vi "HandleObservationSync_002.vi"(8 "error in (no error)":errorcluster, 11 "S4GUI in":refnum<class "S4GUI.lvclass">) -> (0 "error out":errorcluster, 3 "S4GUI out":refnum<class "S4GUI.lvclass">)   [LabVIEW 2018, in "S4GUI.lvclass"] (continued)
          n492 = call-dynamic "Get CCD_Config.vi"("error in (no error)"=w1255, "Interface in"=w1261) -> ("error out"=w1268:errorcluster, "output cluster"=w1270:T1, "Interface out"=w1267:refnum<class "Interface.lvclass">)  [unwired: 7 in]
          n493 = Bundle By Name(cluster=w1270, "TRIGGER_MODE"=w1269) -> (w1266:T1)
          n494 = call-dynamic "Set CCD_Config.vi"("error in (no error)"=w1268, "input cluster"=w1266, "Interface in"=w1267) -> ("error out"=w1264:errorcluster, "Interface out"=w1262:refnum<class "Interface.lvclass">)  [unwired: 7 in]
          n495 = Flatten To String(anything=w1266, error in (no error)=w1264) -> (data string=w1265:string, error out=w1263:errorcluster)  [unwired: 2 in, 1 out]
          n496 = call "Write flatted cluster.vi"("error in (no error)"=w1263, "flatted cluster"=w1265, "Interface in"=w1262) -> ("error out"=w1258:errorcluster, "Interface out"=w1259:refnum<class "Interface.lvclass">)  [unwired: 7 in]
          n497 = Increment(x=w1295) -> (x+1=w1294:u32)
          n498 = call-dynamic "Write Interface.vi"("error in (no error)"=w1258, "Interface.lvclass"=w1259, "Channel in"=w1260) -> ("error out"=w1254:errorcluster, "Channel out"=w1253:refnum<class "Channel.lvclass">)  [unwired: 7 in]
          n499 = call-dynamic "Read State Machine.vi"("error in (no error)"=w1254, "Device in"=w1253) -> ("error out"=w1281:errorcluster, "State Machine.lvclass"=w1283:refnum<class "State Machine.lvclass">, "Device out"=w1279:refnum<class "Channel.lvclass">)  [unwired: 7 in]
          n500 = call "Next State.vi"("error in (no error)"=w1281, "New_State"=60, "State Machine in"=w1283) -> ("error out"=w1276:errorcluster, "State Machine out"=w1277:refnum<class "State Machine.lvclass">)  [unwired: 7 in]
          n501 = call-dynamic "Write State Machine.vi"("error in (no error)"=w1276, "State Machine.lvclass"=w1277, "Device in"=w1279) -> ("error out"=w1278:errorcluster, "Device out"=w1280:refnum<class "Channel.lvclass">)  [unwired: 7 in]
          n502 = call-dynamic "Write Channel.vi"("error in (no error)"=w1278, "Channel.lvclass"=w1280, "Acquisition in"=w1284) -> ("error out"=w1271:errorcluster, "Acquisition out"=w1272:refnum<class "Acquisition.lvclass">)  [unwired: 7 in]
          n503 = call-dynamic "Write AcquisitionA.vi"("error in (no error)"=w1271, "Acquisition.lvclass"=w1272, "S4ACS_GUI in"=w1273) -> ("error out"=w1286:errorcluster, "S4ACS_GUI out"=w1285:refnum<class "S4GUI.lvclass">)  [unwired: 7 in]
          n504 = Bundle By Name(cluster=w1285, "Obs_state"=w1294) -> (w1293:refnum<class "S4GUI.lvclass">)
        }
        frame 254 {
          # "Espera terminar a execução do comando atual \nantes de ir ao proximo passo da Observação."
          n505 = call-dynamic "Read AcquisitionA.vi"("error in (no error)"=w1315, "S4ACS_GUI in"=w1316) -> ("error out"=w1321:errorcluster, "Acquisition.lvclass"=w1322:refnum<class "Acquisition.lvclass">, "S4ACS_GUI out"=w1318:refnum<class "S4GUI.lvclass">)  [unwired: 7 in]
          n506 = call-dynamic "Read Channel.vi"("error in (no error)"=w1321, "Acquisition in"=w1322) -> ("error out"=w1313:errorcluster, "Channel.lvclass"=w1312:refnum<class "Channel.lvclass">, "Acquisition out"=w1320:refnum<class "Acquisition.lvclass">)  [unwired: 7 in]
          n507 = call-dynamic "Read State Machine.vi"("error in (no error)"=w1313, "Device in"=w1312) -> ("error out"=w1304:errorcluster, "State Machine.lvclass"=w1306:refnum<class "State Machine.lvclass">, "Device out"=w1310:refnum<class "Channel.lvclass">)  [unwired: 7 in]
          n508 = call-dynamic "Read State.vi"("error in (no error)"=w1304, "State Machine in"=w1306) -> ("error out"=w1303:errorcluster, "State"=w1300:i32, "State Machine out"=w1305:refnum<class "State Machine.lvclass">)  [unwired: 7 in]
          n509 = Equal To 0?(x=w1300) -> (x = 0?=w1302:bool)
          n510 = call-dynamic "Write State Machine.vi"("error in (no error)"=w1303, "State Machine.lvclass"=w1305, "Device in"=w1310) -> ("error out"=w1309:errorcluster, "Device out"=w1311:refnum<class "Channel.lvclass">)  [unwired: 7 in]
          n511 = call-dynamic "Write Channel.vi"("error in (no error)"=w1309, "Channel.lvclass"=w1311, "Acquisition in"=w1320) -> ("error out"=w1317:errorcluster, "Acquisition out"=w1319:refnum<class "Acquisition.lvclass">)  [unwired: 7 in]
          n512 = disable-structure shown="Enabled" {
            disable-tunnel: [u32 299 ("t") w1324] -> w1299
            disable-tunnel: w1298 -> [_ w1325]
            frame Disabled {
            }
            frame Enabled {
              n513 = Increment(x=w1325) -> (x+1=w1324:u32)
            }
          }
          n514 = Select(t=w1299, s=w1302, f=w1298) -> (s? t:f=w1301:u32)
          n515 = call-dynamic "Write AcquisitionA.vi"("error in (no error)"=w1317, "Acquisition.lvclass"=w1319, "S4ACS_GUI in"=w1318) -> ("error out"=w1314:errorcluster, "S4ACS_GUI out"=w1308:refnum<class "S4GUI.lvclass">)  [unwired: 7 in]
          n516 = Bundle By Name(cluster=w1308, "Obs_state"=w1301) -> (w1307:refnum<class "S4GUI.lvclass">)
        }
        frame 255 {
          n517 = call "Read AcquisitionB.vi"("error in (no error)"=w1336, "S4ACS_GUI in"=w1337) -> ("error out"=w1329:errorcluster, "Acquisition.lvclass"=w1330:refnum<class "Acquisition.lvclass">, "S4ACS_GUI out"=w1339:refnum<class "S4GUI.lvclass">)  [unwired: 7 in]
          n518 = call "Read connection.vi"("error in (no error)"=w1329, "Server in"=w1330) -> ("error out"=w1328:errorcluster, "connection"=w1326:bool, "Server out"=w1327:refnum<class "Acquisition.lvclass">)  [unwired: 7 in]
          n519 = case shown="False" w1326 {
            tunnel: w1327 -> [w1347 w1367]
            tunnel: w1328 -> [w1346 w1366]
            tunnel: [w1347 w1364] -> w1340
            tunnel: [w1346 w1363] -> w1338
            tunnel: w1333 -> [w1345 w1356]
            tunnel: [w1341 w1355] -> w1332
            frame False {
              n520 = Increment(x=w1345) -> (x+1=w1344:u32)
              n521 = Increment(x=w1344) -> (x+1=w1343:u32)
              n522 = Increment(x=w1343) -> (x+1=w1342:u32)
              n523 = Increment(x=w1342) -> (x+1=w1341:u32)
            }
            frame True {
              # "configura o canal,\nmas não dispara\na exposicao."
              n524 = call-dynamic "Read Channel.vi"("error in (no error)"=w1366, "Acquisition in"=w1367) -> ("error out"=w1352:errorcluster, "Channel.lvclass"=w1354:refnum<class "Channel.lvclass">, "Acquisition out"=w1365:refnum<class "Acquisition.lvclass">)  [unwired: 7 in]
              n525 = call-dynamic "Write expose.vi"("error in (no error)"=w1352, "expose"=FALSE, "Channel in"=w1354) -> ("error out"=w1351:errorcluster, "Channel out"=w1353:refnum<class "Channel.lvclass">)  [unwired: 7 in]
              n526 = call-dynamic "Read State Machine.vi"("error in (no error)"=w1351, "Device in"=w1353) -> ("error out"=w1360:errorcluster, "State Machine.lvclass"=w1362:refnum<class "State Machine.lvclass">, "Device out"=w1358:refnum<class "Channel.lvclass">)  [unwired: 7 in]
              n527 = call "Next State.vi"("error in (no error)"=w1360, "New_State"=1, "State Machine in"=w1362) -> ("error out"=w1348:errorcluster, "State Machine out"=w1349:refnum<class "State Machine.lvclass">)  [unwired: 7 in]
              n528 = Increment(x=w1356) -> (x+1=w1355:u32)
              n529 = call-dynamic "Write State Machine.vi"("error in (no error)"=w1348, "State Machine.lvclass"=w1349, "Device in"=w1358) -> ("error out"=w1357:errorcluster, "Device out"=w1359:refnum<class "Channel.lvclass">)  [unwired: 7 in]
              n530 = call-dynamic "Write Channel.vi"("error in (no error)"=w1357, "Channel.lvclass"=w1359, "Acquisition in"=w1365) -> ("error out"=w1363:errorcluster, "Acquisition out"=w1364:refnum<class "Acquisition.lvclass">)  [unwired: 7 in]
            }
          }
          n531 = call "Write AcquisitionB.vi"("error in (no error)"=w1338, "Acquisition.lvclass"=w1340, "S4ACS_GUI in"=w1339) -> ("error out"=w1335:errorcluster, "S4ACS_GUI out"=w1334:refnum<class "S4GUI.lvclass">)  [unwired: 7 in]
          n532 = Bundle By Name(cluster=w1334, "Obs_state"=w1332) -> (w1331:refnum<class "S4GUI.lvclass">)
        }
        frame 256 {
          # "Espera terminar a execução do comando atual \nantes de ir ao proximo passo da Observação."
          n533 = call "Read AcquisitionB.vi"("error in (no error)"=w1385, "S4ACS_GUI in"=w1386) -> ("error out"=w1391:errorcluster, "Acquisition.lvclass"=w1392:refnum<class "Acquisition.lvclass">, "S4ACS_GUI out"=w1388:refnum<class "S4GUI.lvclass">)  [unwired: 7 in]
          n534 = call-dynamic "Read Channel.vi"("error in (no error)"=w1391, "Acquisition in"=w1392) -> ("error out"=w1383:errorcluster, "Channel.lvclass"=w1382:refnum<class "Channel.lvclass">, "Acquisition out"=w1390:refnum<class "Acquisition.lvclass">)  [unwired: 7 in]
          n535 = call-dynamic "Read State Machine.vi"("error in (no error)"=w1383, "Device in"=w1382) -> ("error out"=w1374:errorcluster, "State Machine.lvclass"=w1376:refnum<class "State Machine.lvclass">, "Device out"=w1380:refnum<class "Channel.lvclass">)  [unwired: 7 in]
          n536 = call-dynamic "Read State.vi"("error in (no error)"=w1374, "State Machine in"=w1376) -> ("error out"=w1373:errorcluster, "State"=w1370:i32, "State Machine out"=w1375:refnum<class "State Machine.lvclass">)  [unwired: 7 in]
          n537 = call-dynamic "Write State Machine.vi"("error in (no error)"=w1373, "State Machine.lvclass"=w1375, "Device in"=w1380) -> ("error out"=w1379:errorcluster, "Device out"=w1381:refnum<class "Channel.lvclass">)  [unwired: 7 in]
          n538 = call-dynamic "Write Channel.vi"("error in (no error)"=w1379, "Channel.lvclass"=w1381, "Acquisition in"=w1390) -> ("error out"=w1387:errorcluster, "Acquisition out"=w1389:refnum<class "Acquisition.lvclass">)  [unwired: 7 in]
          n539 = Equal To 0?(x=w1370) -> (x = 0?=w1372:bool)
          n540 = disable-structure shown="Enabled" {
            disable-tunnel: [u32 299 ("t") w1394] -> w1368
            disable-tunnel: w1369 -> [_ w1397]
            frame Disabled {
            }
            frame Enabled {
              n541 = Increment(x=w1397) -> (x+1=w1396:u32)
              n542 = Increment(x=w1396) -> (x+1=w1395:u32)
              n543 = Increment(x=w1395) -> (x+1=w1394:u32)
            }
          }
          n544 = Select(t=w1368, s=w1372, f=w1369) -> (s? t:f=w1371:u32)
          n545 = call "Write AcquisitionB.vi"("error in (no error)"=w1387, "Acquisition.lvclass"=w1389, "S4ACS_GUI in"=w1388) -> ("error out"=w1384:errorcluster, "S4ACS_GUI out"=w1378:refnum<class "S4GUI.lvclass">)  [unwired: 7 in]
          n546 = Bundle By Name(cluster=w1378, "Obs_state"=w1371) -> (w1377:refnum<class "S4GUI.lvclass">)
        }
        frame 257 {
          # "Sem SyncBox, \ntrigger mode = 0 (internal)\nCom SyncBox\ntrigger mode = 6 (ext. start)"
          n547 = call-dynamic "Read Sync Box.lvclass.vi"("error in (no error)"=w1435, "SPARC4_AC in"=w1434) -> ("error out"=w1437:errorcluster, "Sync Box.lvclass"=w1438:refnum<class "Sync Box.lvclass">, "SPARC4_AC out"=w1433:refnum<class "S4GUI.lvclass">)  [unwired: 7 in]
          n548 = call "Read connection.vi"("error in (no error)"=w1437, "Server in"=w1438) -> ("error out"=w1436:errorcluster, "connection"=w1399:bool)  [unwired: 7 in, 1 out]
          n549 = case shown="False" w1399 {
            tunnel: [u8 6 ("TRIGGER_MODE") u8 0 ("TRIGGER_MODE")] -> w1398
            frame True {
            }
            frame False {
            }
          }
          n550 = call "Read AcquisitionB.vi"("error in (no error)"=w1436, "S4ACS_GUI in"=w1433) -> ("error out"=w1420:errorcluster, "Acquisition.lvclass"=w1421:refnum<class "Acquisition.lvclass">, "S4ACS_GUI out"=w1419:refnum<class "S4GUI.lvclass">)  [unwired: 7 in]
          n551 = call-dynamic "Read Channel.vi"("error in (no error)"=w1420, "Acquisition in"=w1421) -> ("error out"=w1404:errorcluster, "Channel.lvclass"=w1403:refnum<class "Channel.lvclass">, "Acquisition out"=w1430:refnum<class "Acquisition.lvclass">)  [unwired: 7 in]
          n552 = call-dynamic "Read Interface.vi"("error in (no error)"=w1404, "Channel in"=w1403) -> ("error out"=w1402:errorcluster, "Interface.lvclass"=w1408:refnum<class "Interface.lvclass">, "Channel out"=w1407:refnum<class "Channel.lvclass">)  [unwired: 7 in]
          n553 = call-dynamic "Get CCD_Config.vi"("error in (no error)"=w1402, "Interface in"=w1408) -> ("error out"=w1415:errorcluster, "output cluster"=w1416:T1, "Interface out"=w1414:refnum<class "Interface.lvclass">)  [unwired: 7 in]
          n554 = Bundle By Name(cluster=w1416, "TRIGGER_MODE"=w1398) -> (w1413:T1)
          n555 = call-dynamic "Set CCD_Config.vi"("error in (no error)"=w1415, "input cluster"=w1413, "Interface in"=w1414) -> ("error out"=w1411:errorcluster, "Interface out"=w1409:refnum<class "Interface.lvclass">)  [unwired: 7 in]
          n556 = Flatten To String(anything=w1413, error in (no error)=w1411) -> (data string=w1412:string, error out=w1410:errorcluster)  [unwired: 2 in, 1 out]
          n557 = call "Write flatted cluster.vi"("error in (no error)"=w1410, "flatted cluster"=w1412, "Interface in"=w1409) -> ("error out"=w1405:errorcluster, "Interface out"=w1406:refnum<class "Interface.lvclass">)  [unwired: 7 in]
          n558 = Increment(x=w1441) -> (x+1=w1440:u32)
          n559 = call-dynamic "Write Interface.vi"("error in (no error)"=w1405, "Interface.lvclass"=w1406, "Channel in"=w1407) -> ("error out"=w1401:errorcluster, "Channel out"=w1400:refnum<class "Channel.lvclass">)  [unwired: 7 in]
          n560 = call-dynamic "Read State Machine.vi"("error in (no error)"=w1401, "Device in"=w1400) -> ("error out"=w1427:errorcluster, "State Machine.lvclass"=w1429:refnum<class "State Machine.lvclass">, "Device out"=w1425:refnum<class "Channel.lvclass">)  [unwired: 7 in]
          n561 = call "Next State.vi"("error in (no error)"=w1427, "New_State"=60, "State Machine in"=w1429) -> ("error out"=w1422:errorcluster, "State Machine out"=w1423:refnum<class "State Machine.lvclass">)  [unwired: 7 in]
          n562 = call-dynamic "Write State Machine.vi"("error in (no error)"=w1422, "State Machine.lvclass"=w1423, "Device in"=w1425) -> ("error out"=w1424:errorcluster, "Device out"=w1426:refnum<class "Channel.lvclass">)  [unwired: 7 in]
          n563 = call-dynamic "Write Channel.vi"("error in (no error)"=w1424, "Channel.lvclass"=w1426, "Acquisition in"=w1430) -> ("error out"=w1417:errorcluster, "Acquisition out"=w1418:refnum<class "Acquisition.lvclass">)  [unwired: 7 in]
          n564 = call "Write AcquisitionB.vi"("error in (no error)"=w1417, "Acquisition.lvclass"=w1418, "S4ACS_GUI in"=w1419) -> ("error out"=w1432:errorcluster, "S4ACS_GUI out"=w1431:refnum<class "S4GUI.lvclass">)  [unwired: 7 in]
          n565 = Bundle By Name(cluster=w1431, "Obs_state"=w1440) -> (w1439:refnum<class "S4GUI.lvclass">)
        }
        frame 258 {
          # "Espera terminar a execução do comando atual \nantes de ir ao proximo passo da Observação."
          n566 = call "Read AcquisitionB.vi"("error in (no error)"=w1461, "S4ACS_GUI in"=w1462) -> ("error out"=w1467:errorcluster, "Acquisition.lvclass"=w1468:refnum<class "Acquisition.lvclass">, "S4ACS_GUI out"=w1464:refnum<class "S4GUI.lvclass">)  [unwired: 7 in]
          n567 = call-dynamic "Read Channel.vi"("error in (no error)"=w1467, "Acquisition in"=w1468) -> ("error out"=w1459:errorcluster, "Channel.lvclass"=w1458:refnum<class "Channel.lvclass">, "Acquisition out"=w1466:refnum<class "Acquisition.lvclass">)  [unwired: 7 in]
          n568 = call-dynamic "Read State Machine.vi"("error in (no error)"=w1459, "Device in"=w1458) -> ("error out"=w1450:errorcluster, "State Machine.lvclass"=w1452:refnum<class "State Machine.lvclass">, "Device out"=w1456:refnum<class "Channel.lvclass">)  [unwired: 7 in]
          n569 = call-dynamic "Read State.vi"("error in (no error)"=w1450, "State Machine in"=w1452) -> ("error out"=w1449:errorcluster, "State"=w1446:i32, "State Machine out"=w1451:refnum<class "State Machine.lvclass">)  [unwired: 7 in]
          n570 = call-dynamic "Write State Machine.vi"("error in (no error)"=w1449, "State Machine.lvclass"=w1451, "Device in"=w1456) -> ("error out"=w1455:errorcluster, "Device out"=w1457:refnum<class "Channel.lvclass">)  [unwired: 7 in]
          n571 = call-dynamic "Write Channel.vi"("error in (no error)"=w1455, "Channel.lvclass"=w1457, "Acquisition in"=w1466) -> ("error out"=w1463:errorcluster, "Acquisition out"=w1465:refnum<class "Acquisition.lvclass">)  [unwired: 7 in]
          n572 = Equal To 0?(x=w1446) -> (x = 0?=w1448:bool)
          n573 = Increment(x=w1445) -> (x+1=w1444:u32)
          n574 = Select(t=w1444, s=w1448, f=w1445) -> (s? t:f=w1447:u32)
          n575 = call "Write AcquisitionB.vi"("error in (no error)"=w1463, "Acquisition.lvclass"=w1465, "S4ACS_GUI in"=w1464) -> ("error out"=w1460:errorcluster, "S4ACS_GUI out"=w1454:refnum<class "S4GUI.lvclass">)  [unwired: 7 in]
          n576 = Bundle By Name(cluster=w1454, "Obs_state"=w1447) -> (w1453:refnum<class "S4GUI.lvclass">)
        }
        frame 259 {
          n577 = call-dynamic "Read AcquisitionC.vi"("error in (no error)"=w1479, "S4ACS_GUI in"=w1480) -> ("error out"=w1471:errorcluster, "Acquisition.lvclass"=w1473:refnum<class "Acquisition.lvclass">, "S4ACS_GUI out"=w1482:refnum<class "S4GUI.lvclass">)  [unwired: 7 in]
          n578 = call "Read connection.vi"("error in (no error)"=w1471, "Server in"=w1473) -> ("error out"=w1470:errorcluster, "connection"=w1469:bool, "Server out"=w1472:refnum<class "Acquisition.lvclass">)  [unwired: 7 in]
          n579 = case shown="True" w1469 {
            tunnel: w1472 -> [w1489 w1510]
            tunnel: w1470 -> [w1490 w1509]
            tunnel: [w1489 w1507] -> w1483
            tunnel: [w1490 w1506] -> w1481
            tunnel: w1476 -> [w1488 w1499]
            tunnel: [w1484 w1498] -> w1475
            frame False {
              n580 = Increment(x=w1488) -> (x+1=w1487:u32)
              n581 = Increment(x=w1487) -> (x+1=w1486:u32)
              n582 = Increment(x=w1486) -> (x+1=w1485:u32)
              n583 = Increment(x=w1485) -> (x+1=w1484:u32)
            }
            frame True {
              # "configura o canal,\nmas não dispara\na exposicao."
              n584 = call-dynamic "Read Channel.vi"("error in (no error)"=w1509, "Acquisition in"=w1510) -> ("error out"=w1495:errorcluster, "Channel.lvclass"=w1497:refnum<class "Channel.lvclass">, "Acquisition out"=w1508:refnum<class "Acquisition.lvclass">)  [unwired: 7 in]
              n585 = call-dynamic "Write expose.vi"("error in (no error)"=w1495, "expose"=FALSE, "Channel in"=w1497) -> ("error out"=w1494:errorcluster, "Channel out"=w1496:refnum<class "Channel.lvclass">)  [unwired: 7 in]
              n586 = call-dynamic "Read State Machine.vi"("error in (no error)"=w1494, "Device in"=w1496) -> ("error out"=w1503:errorcluster, "State Machine.lvclass"=w1505:refnum<class "State Machine.lvclass">, "Device out"=w1501:refnum<class "Channel.lvclass">)  [unwired: 7 in]
              n587 = call "Next State.vi"("error in (no error)"=w1503, "New_State"=1, "State Machine in"=w1505) -> ("error out"=w1491:errorcluster, "State Machine out"=w1492:refnum<class "State Machine.lvclass">)  [unwired: 7 in]
              n588 = Increment(x=w1499) -> (x+1=w1498:u32)
              n589 = call-dynamic "Write State Machine.vi"("error in (no error)"=w1491, "State Machine.lvclass"=w1492, "Device in"=w1501) -> ("error out"=w1500:errorcluster, "Device out"=w1502:refnum<class "Channel.lvclass">)  [unwired: 7 in]
              n590 = call-dynamic "Write Channel.vi"("error in (no error)"=w1500, "Channel.lvclass"=w1502, "Acquisition in"=w1508) -> ("error out"=w1506:errorcluster, "Acquisition out"=w1507:refnum<class "Acquisition.lvclass">)  [unwired: 7 in]
            }
          }
          n591 = call-dynamic "Write AcquisitionC.vi"("error in (no error)"=w1481, "Acquisition.lvclass"=w1483, "S4ACS_GUI in"=w1482) -> ("error out"=w1478:errorcluster, "S4ACS_GUI out"=w1477:refnum<class "S4GUI.lvclass">)  [unwired: 7 in]
          n592 = Bundle By Name(cluster=w1477, "Obs_state"=w1475) -> (w1474:refnum<class "S4GUI.lvclass">)
        }
        frame 260 {
          # "Espera terminar a execução do comando atual \nantes de ir ao proximo passo da Observação."
          n593 = call-dynamic "Read AcquisitionC.vi"("error in (no error)"=w1528, "S4ACS_GUI in"=w1529) -> ("error out"=w1534:errorcluster, "Acquisition.lvclass"=w1535:refnum<class "Acquisition.lvclass">, "S4ACS_GUI out"=w1531:refnum<class "S4GUI.lvclass">)  [unwired: 7 in]
          n594 = call-dynamic "Read Channel.vi"("error in (no error)"=w1534, "Acquisition in"=w1535) -> ("error out"=w1526:errorcluster, "Channel.lvclass"=w1525:refnum<class "Channel.lvclass">, "Acquisition out"=w1533:refnum<class "Acquisition.lvclass">)  [unwired: 7 in]
          n595 = call-dynamic "Read State Machine.vi"("error in (no error)"=w1526, "Device in"=w1525) -> ("error out"=w1517:errorcluster, "State Machine.lvclass"=w1519:refnum<class "State Machine.lvclass">, "Device out"=w1523:refnum<class "Channel.lvclass">)  [unwired: 7 in]
          n596 = call-dynamic "Read State.vi"("error in (no error)"=w1517, "State Machine in"=w1519) -> ("error out"=w1516:errorcluster, "State"=w1513:i32, "State Machine out"=w1518:refnum<class "State Machine.lvclass">)  [unwired: 7 in]
          n597 = Equal To 0?(x=w1513) -> (x = 0?=w1515:bool)
          n598 = call-dynamic "Write State Machine.vi"("error in (no error)"=w1516, "State Machine.lvclass"=w1518, "Device in"=w1523) -> ("error out"=w1522:errorcluster, "Device out"=w1524:refnum<class "Channel.lvclass">)  [unwired: 7 in]
          n599 = call-dynamic "Write Channel.vi"("error in (no error)"=w1522, "Channel.lvclass"=w1524, "Acquisition in"=w1533) -> ("error out"=w1530:errorcluster, "Acquisition out"=w1532:refnum<class "Acquisition.lvclass">)  [unwired: 7 in]
          n600 = disable-structure shown="Enabled" {
            disable-tunnel: [u32 299 ("t") w1537] -> w1511
            disable-tunnel: w1512 -> [_ w1540]
            frame Disabled {
            }
            frame Enabled {
              n601 = Increment(x=w1540) -> (x+1=w1539:u32)
              n602 = Increment(x=w1539) -> (x+1=w1538:u32)
              n603 = Increment(x=w1538) -> (x+1=w1537:u32)
            }
          }
          n604 = Select(t=w1511, s=w1515, f=w1512) -> (s? t:f=w1514:u32)
          n605 = call-dynamic "Write AcquisitionC.vi"("error in (no error)"=w1530, "Acquisition.lvclass"=w1532, "S4ACS_GUI in"=w1531) -> ("error out"=w1527:errorcluster, "S4ACS_GUI out"=w1521:refnum<class "S4GUI.lvclass">)  [unwired: 7 in]
          n606 = Bundle By Name(cluster=w1521, "Obs_state"=w1514) -> (w1520:refnum<class "S4GUI.lvclass">)
        }
        frame 261 {
          # "Sem SyncBox, \ntrigger mode = 0 (internal)\nCom SyncBox\ntrigger mode = 6 (ext. start)"
          n607 = call-dynamic "Read Sync Box.lvclass.vi"("error in (no error)"=w1578, "SPARC4_AC in"=w1577) -> ("error out"=w1580:errorcluster, "Sync Box.lvclass"=w1581:refnum<class "Sync Box.lvclass">, "SPARC4_AC out"=w1576:refnum<class "S4GUI.lvclass">)  [unwired: 7 in]
          n608 = call "Read connection.vi"("error in (no error)"=w1580, "Server in"=w1581) -> ("error out"=w1579:errorcluster, "connection"=w1542:bool)  [unwired: 7 in, 1 out]
          n609 = case shown="False" w1542 {
            tunnel: [u8 6 ("TRIGGER_MODE") u8 0 ("TRIGGER_MODE")] -> w1541
            frame True {
            }
            frame False {
            }
          }
          n610 = call-dynamic "Read AcquisitionC.vi"("error in (no error)"=w1579, "S4ACS_GUI in"=w1576) -> ("error out"=w1563:errorcluster, "Acquisition.lvclass"=w1564:refnum<class "Acquisition.lvclass">, "S4ACS_GUI out"=w1562:refnum<class "S4GUI.lvclass">)  [unwired: 7 in]
          n611 = call-dynamic "Read Channel.vi"("error in (no error)"=w1563, "Acquisition in"=w1564) -> ("error out"=w1547:errorcluster, "Channel.lvclass"=w1546:refnum<class "Channel.lvclass">, "Acquisition out"=w1573:refnum<class "Acquisition.lvclass">)  [unwired: 7 in]
          n612 = call-dynamic "Read Interface.vi"("error in (no error)"=w1547, "Channel in"=w1546) -> ("error out"=w1545:errorcluster, "Interface.lvclass"=w1551:refnum<class "Interface.lvclass">, "Channel out"=w1550:refnum<class "Channel.lvclass">)  [unwired: 7 in]
          n613 = call-dynamic "Get CCD_Config.vi"("error in (no error)"=w1545, "Interface in"=w1551) -> ("error out"=w1558:errorcluster, "output cluster"=w1559:T1, "Interface out"=w1557:refnum<class "Interface.lvclass">)  [unwired: 7 in]
          n614 = Bundle By Name(cluster=w1559, "TRIGGER_MODE"=w1541) -> (w1556:T1)
          n615 = call-dynamic "Set CCD_Config.vi"("error in (no error)"=w1558, "input cluster"=w1556, "Interface in"=w1557) -> ("error out"=w1554:errorcluster, "Interface out"=w1552:refnum<class "Interface.lvclass">)  [unwired: 7 in]
          n616 = Flatten To String(anything=w1556, error in (no error)=w1554) -> (data string=w1555:string, error out=w1553:errorcluster)  [unwired: 2 in, 1 out]
          n617 = call "Write flatted cluster.vi"("error in (no error)"=w1553, "flatted cluster"=w1555, "Interface in"=w1552) -> ("error out"=w1548:errorcluster, "Interface out"=w1549:refnum<class "Interface.lvclass">)  [unwired: 7 in]
          n618 = Increment(x=w1584) -> (x+1=w1583:u32)
          n619 = call-dynamic "Write Interface.vi"("error in (no error)"=w1548, "Interface.lvclass"=w1549, "Channel in"=w1550) -> ("error out"=w1544:errorcluster, "Channel out"=w1543:refnum<class "Channel.lvclass">)  [unwired: 7 in]
          n620 = call-dynamic "Read State Machine.vi"("error in (no error)"=w1544, "Device in"=w1543) -> ("error out"=w1570:errorcluster, "State Machine.lvclass"=w1572:refnum<class "State Machine.lvclass">, "Device out"=w1568:refnum<class "Channel.lvclass">)  [unwired: 7 in]
          n621 = call "Next State.vi"("error in (no error)"=w1570, "New_State"=60, "State Machine in"=w1572) -> ("error out"=w1565:errorcluster, "State Machine out"=w1566:refnum<class "State Machine.lvclass">)  [unwired: 7 in]
          n622 = call-dynamic "Write State Machine.vi"("error in (no error)"=w1565, "State Machine.lvclass"=w1566, "Device in"=w1568) -> ("error out"=w1567:errorcluster, "Device out"=w1569:refnum<class "Channel.lvclass">)  [unwired: 7 in]
          n623 = call-dynamic "Write Channel.vi"("error in (no error)"=w1567, "Channel.lvclass"=w1569, "Acquisition in"=w1573) -> ("error out"=w1560:errorcluster, "Acquisition out"=w1561:refnum<class "Acquisition.lvclass">)  [unwired: 7 in]
          n624 = call-dynamic "Write AcquisitionC.vi"("error in (no error)"=w1560, "Acquisition.lvclass"=w1561, "S4ACS_GUI in"=w1562) -> ("error out"=w1575:errorcluster, "S4ACS_GUI out"=w1574:refnum<class "S4GUI.lvclass">)  [unwired: 7 in]
          n625 = Bundle By Name(cluster=w1574, "Obs_state"=w1583) -> (w1582:refnum<class "S4GUI.lvclass">)
        }
        frame 262 {
          # "Espera terminar a execução do comando atual \nantes de ir ao proximo passo da Observação."
          n626 = call-dynamic "Read AcquisitionC.vi"("error in (no error)"=w1604, "S4ACS_GUI in"=w1605) -> ("error out"=w1610:errorcluster, "Acquisition.lvclass"=w1611:refnum<class "Acquisition.lvclass">, "S4ACS_GUI out"=w1607:refnum<class "S4GUI.lvclass">)  [unwired: 7 in]
          n627 = call-dynamic "Read Channel.vi"("error in (no error)"=w1610, "Acquisition in"=w1611) -> ("error out"=w1602:errorcluster, "Channel.lvclass"=w1601:refnum<class "Channel.lvclass">, "Acquisition out"=w1609:refnum<class "Acquisition.lvclass">)  [unwired: 7 in]
          n628 = call-dynamic "Read State Machine.vi"("error in (no error)"=w1602, "Device in"=w1601) -> ("error out"=w1593:errorcluster, "State Machine.lvclass"=w1595:refnum<class "State Machine.lvclass">, "Device out"=w1599:refnum<class "Channel.lvclass">)  [unwired: 7 in]
          n629 = call-dynamic "Read State.vi"("error in (no error)"=w1593, "State Machine in"=w1595) -> ("error out"=w1592:errorcluster, "State"=w1589:i32, "State Machine out"=w1594:refnum<class "State Machine.lvclass">)  [unwired: 7 in]
          n630 = Equal To 0?(x=w1589) -> (x = 0?=w1591:bool)
          n631 = call-dynamic "Write State Machine.vi"("error in (no error)"=w1592, "State Machine.lvclass"=w1594, "Device in"=w1599) -> ("error out"=w1598:errorcluster, "Device out"=w1600:refnum<class "Channel.lvclass">)  [unwired: 7 in]
          n632 = call-dynamic "Write Channel.vi"("error in (no error)"=w1598, "Channel.lvclass"=w1600, "Acquisition in"=w1609) -> ("error out"=w1606:errorcluster, "Acquisition out"=w1608:refnum<class "Acquisition.lvclass">)  [unwired: 7 in]
          n633 = Increment(x=w1588) -> (x+1=w1587:u32)
          n634 = Select(t=w1587, s=w1591, f=w1588) -> (s? t:f=w1590:u32)
          n635 = call-dynamic "Write AcquisitionC.vi"("error in (no error)"=w1606, "Acquisition.lvclass"=w1608, "S4ACS_GUI in"=w1607) -> ("error out"=w1603:errorcluster, "S4ACS_GUI out"=w1597:refnum<class "S4GUI.lvclass">)  [unwired: 7 in]
          n636 = Bundle By Name(cluster=w1597, "Obs_state"=w1590) -> (w1596:refnum<class "S4GUI.lvclass">)
        }
        frame 263 {
          # "Dispara o comando para o dispositivo corrente."
          n637 = call-dynamic "Read AcquisitionD.vi"("error in (no error)"=w1622, "S4ACS_GUI in"=w1623) -> ("error out"=w1615:errorcluster, "Acquisition.lvclass"=w1616:refnum<class "Acquisition.lvclass">, "S4ACS_GUI out"=w1625:refnum<class "S4GUI.lvclass">)  [unwired: 7 in]
          n638 = call "Read connection.vi"("error in (no error)"=w1615, "Server in"=w1616) -> ("error out"=w1613:errorcluster, "connection"=w1612:bool, "Server out"=w1614:refnum<class "Acquisition.lvclass">)  [unwired: 7 in]
          n639 = case shown="True" w1612 {
            tunnel: w1614 -> [w1629 w1649]
            tunnel: w1613 -> [w1628 w1648]
            tunnel: [w1629 w1646] -> w1626
            tunnel: [w1628 w1645] -> w1624
            tunnel: w1619 -> [_ w1638]
            tunnel: [u32 299 w1637] -> w1618
            frame False {
            }
            frame True {
              # "configura o canal,\nmas não dispara\na exposicao."
              n640 = call-dynamic "Read Channel.vi"("error in (no error)"=w1648, "Acquisition in"=w1649) -> ("error out"=w1634:errorcluster, "Channel.lvclass"=w1636:refnum<class "Channel.lvclass">, "Acquisition out"=w1647:refnum<class "Acquisition.lvclass">)  [unwired: 7 in]
              n641 = call-dynamic "Write expose.vi"("error in (no error)"=w1634, "expose"=FALSE, "Channel in"=w1636) -> ("error out"=w1633:errorcluster, "Channel out"=w1635:refnum<class "Channel.lvclass">)  [unwired: 7 in]
              n642 = call-dynamic "Read State Machine.vi"("error in (no error)"=w1633, "Device in"=w1635) -> ("error out"=w1642:errorcluster, "State Machine.lvclass"=w1644:refnum<class "State Machine.lvclass">, "Device out"=w1640:refnum<class "Channel.lvclass">)  [unwired: 7 in]
              n643 = call "Next State.vi"("error in (no error)"=w1642, "New_State"=1, "State Machine in"=w1644) -> ("error out"=w1630:errorcluster, "State Machine out"=w1631:refnum<class "State Machine.lvclass">)  [unwired: 7 in]
              n644 = Increment(x=w1638) -> (x+1=w1637:u32)
              n645 = call-dynamic "Write State Machine.vi"("error in (no error)"=w1630, "State Machine.lvclass"=w1631, "Device in"=w1640) -> ("error out"=w1639:errorcluster, "Device out"=w1641:refnum<class "Channel.lvclass">)  [unwired: 7 in]
              n646 = call-dynamic "Write Channel.vi"("error in (no error)"=w1639, "Channel.lvclass"=w1641, "Acquisition in"=w1647) -> ("error out"=w1645:errorcluster, "Acquisition out"=w1646:refnum<class "Acquisition.lvclass">)  [unwired: 7 in]
            }
          }
          n647 = call-dynamic "Write AcquisitionD.vi"("error in (no error)"=w1624, "Acquisition.lvclass"=w1626, "S4ACS_GUI in"=w1625) -> ("error out"=w1621:errorcluster, "S4ACS_GUI out"=w1620:refnum<class "S4GUI.lvclass">)  [unwired: 7 in]
          n648 = Bundle By Name(cluster=w1620, "Obs_state"=w1618) -> (w1617:refnum<class "S4GUI.lvclass">)
        }
        frame 264 {
          # "Espera terminar a execução do comando atual \nantes de ir ao proximo passo da Observação."
          n649 = call-dynamic "Read AcquisitionD.vi"("error in (no error)"=w1667, "S4ACS_GUI in"=w1668) -> ("error out"=w1673:errorcluster, "Acquisition.lvclass"=w1674:refnum<class "Acquisition.lvclass">, "S4ACS_GUI out"=w1670:refnum<class "S4GUI.lvclass">)  [unwired: 7 in]
          n650 = call-dynamic "Read Channel.vi"("error in (no error)"=w1673, "Acquisition in"=w1674) -> ("error out"=w1665:errorcluster, "Channel.lvclass"=w1664:refnum<class "Channel.lvclass">, "Acquisition out"=w1672:refnum<class "Acquisition.lvclass">)  [unwired: 7 in]
          n651 = call-dynamic "Read State Machine.vi"("error in (no error)"=w1665, "Device in"=w1664) -> ("error out"=w1656:errorcluster, "State Machine.lvclass"=w1658:refnum<class "State Machine.lvclass">, "Device out"=w1662:refnum<class "Channel.lvclass">)  [unwired: 7 in]
          n652 = call-dynamic "Read State.vi"("error in (no error)"=w1656, "State Machine in"=w1658) -> ("error out"=w1655:errorcluster, "State"=w1652:i32, "State Machine out"=w1657:refnum<class "State Machine.lvclass">)  [unwired: 7 in]
          n653 = Equal To 0?(x=w1652) -> (x = 0?=w1654:bool)
          n654 = call-dynamic "Write State Machine.vi"("error in (no error)"=w1655, "State Machine.lvclass"=w1657, "Device in"=w1662) -> ("error out"=w1661:errorcluster, "Device out"=w1663:refnum<class "Channel.lvclass">)  [unwired: 7 in]
          n655 = call-dynamic "Write Channel.vi"("error in (no error)"=w1661, "Channel.lvclass"=w1663, "Acquisition in"=w1672) -> ("error out"=w1669:errorcluster, "Acquisition out"=w1671:refnum<class "Acquisition.lvclass">)  [unwired: 7 in]
          n656 = disable-structure shown="Enabled" {
            disable-tunnel: w1651 -> [w1676 _]
            disable-tunnel: [w1675 u32 299] -> w1650
            frame Disabled {
              n657 = Increment(x=w1676) -> (x+1=w1675:u32)
            }
            frame Enabled {
            }
          }
          n658 = Select(t=w1650, s=w1654, f=w1651) -> (s? t:f=w1653:u32)
          n659 = call-dynamic "Write AcquisitionD.vi"("error in (no error)"=w1669, "Acquisition.lvclass"=w1671, "S4ACS_GUI in"=w1670) -> ("error out"=w1666:errorcluster, "S4ACS_GUI out"=w1660:refnum<class "S4GUI.lvclass">)  [unwired: 7 in]
          n660 = Bundle By Name(cluster=w1660, "Obs_state"=w1653) -> (w1659:refnum<class "S4GUI.lvclass">)
        }
        frame 265 {
          # "Sem SyncBox, \ntrigger mode = 0 (internal)\nCom SyncBox\ntrigger mode = 6 (ext. start)"
          n661 = call-dynamic "Read Sync Box.lvclass.vi"("error in (no error)"=w1715, "SPARC4_AC in"=w1714) -> ("error out"=w1717:errorcluster, "Sync Box.lvclass"=w1718:refnum<class "Sync Box.lvclass">, "SPARC4_AC out"=w1713:refnum<class "S4GUI.lvclass">)  [unwired: 7 in]
          n662 = call "Read connection.vi"("error in (no error)"=w1717, "Server in"=w1718) -> ("error out"=w1716:errorcluster, "connection"=w1679:bool)  [unwired: 7 in, 1 out]
          n663 = case shown="False" w1679 {
            tunnel: [u8 6 ("TRIGGER_MODE") u8 0 ("TRIGGER_MODE")] -> w1678
            frame True {
            }
            frame False {
            }
          }
          n664 = call-dynamic "Read AcquisitionD.vi"("error in (no error)"=w1716, "S4ACS_GUI in"=w1713) -> ("error out"=w1700:errorcluster, "Acquisition.lvclass"=w1701:refnum<class "Acquisition.lvclass">, "S4ACS_GUI out"=w1699:refnum<class "S4GUI.lvclass">)  [unwired: 7 in]
          n665 = call-dynamic "Read Channel.vi"("error in (no error)"=w1700, "Acquisition in"=w1701) -> ("error out"=w1684:errorcluster, "Channel.lvclass"=w1683:refnum<class "Channel.lvclass">, "Acquisition out"=w1710:refnum<class "Acquisition.lvclass">)  [unwired: 7 in]
          n666 = call-dynamic "Read Interface.vi"("error in (no error)"=w1684, "Channel in"=w1683) -> ("error out"=w1682:errorcluster, "Interface.lvclass"=w1688:refnum<class "Interface.lvclass">, "Channel out"=w1687:refnum<class "Channel.lvclass">)  [unwired: 7 in]
          n667 = call-dynamic "Get CCD_Config.vi"("error in (no error)"=w1682, "Interface in"=w1688) -> ("error out"=w1695:errorcluster, "output cluster"=w1696:T1, "Interface out"=w1694:refnum<class "Interface.lvclass">)  [unwired: 7 in]
          n668 = Bundle By Name(cluster=w1696, "TRIGGER_MODE"=w1678) -> (w1693:T1)
          n669 = call-dynamic "Set CCD_Config.vi"("error in (no error)"=w1695, "input cluster"=w1693, "Interface in"=w1694) -> ("error out"=w1691:errorcluster, "Interface out"=w1689:refnum<class "Interface.lvclass">)  [unwired: 7 in]
          n670 = Flatten To String(anything=w1693, error in (no error)=w1691) -> (data string=w1692:string, error out=w1690:errorcluster)  [unwired: 2 in, 1 out]
          n671 = call "Write flatted cluster.vi"("error in (no error)"=w1690, "flatted cluster"=w1692, "Interface in"=w1689) -> ("error out"=w1685:errorcluster, "Interface out"=w1686:refnum<class "Interface.lvclass">)  [unwired: 7 in]
          n672 = call-dynamic "Write Interface.vi"("error in (no error)"=w1685, "Interface.lvclass"=w1686, "Channel in"=w1687) -> ("error out"=w1681:errorcluster, "Channel out"=w1680:refnum<class "Channel.lvclass">)  [unwired: 7 in]
          n673 = call-dynamic "Read State Machine.vi"("error in (no error)"=w1681, "Device in"=w1680) -> ("error out"=w1707:errorcluster, "State Machine.lvclass"=w1709:refnum<class "State Machine.lvclass">, "Device out"=w1705:refnum<class "Channel.lvclass">)  [unwired: 7 in]
          n674 = Increment(x=w1721) -> (x+1=w1720:u32)
          n675 = call "Next State.vi"("error in (no error)"=w1707, "New_State"=60, "State Machine in"=w1709) -> ("error out"=w1702:errorcluster, "State Machine out"=w1703:refnum<class "State Machine.lvclass">)  [unwired: 7 in]
          n676 = call-dynamic "Write State Machine.vi"("error in (no error)"=w1702, "State Machine.lvclass"=w1703, "Device in"=w1705) -> ("error out"=w1704:errorcluster, "Device out"=w1706:refnum<class "Channel.lvclass">)  [unwired: 7 in]
          n677 = call-dynamic "Write Channel.vi"("error in (no error)"=w1704, "Channel.lvclass"=w1706, "Acquisition in"=w1710) -> ("error out"=w1697:errorcluster, "Acquisition out"=w1698:refnum<class "Acquisition.lvclass">)  [unwired: 7 in]
          n678 = call-dynamic "Write AcquisitionD.vi"("error in (no error)"=w1697, "Acquisition.lvclass"=w1698, "S4ACS_GUI in"=w1699) -> ("error out"=w1712:errorcluster, "S4ACS_GUI out"=w1711:refnum<class "S4GUI.lvclass">)  [unwired: 7 in]
          n679 = Bundle By Name(cluster=w1711, "Obs_state"=w1720) -> (w1719:refnum<class "S4GUI.lvclass">)
        }
        frame 266 {
          # "Espera terminar a execução do comando atual \nantes de ir ao proximo passo da Observação."
          n680 = call-dynamic "Read AcquisitionD.vi"("error in (no error)"=w1741, "S4ACS_GUI in"=w1742) -> ("error out"=w1747:errorcluster, "Acquisition.lvclass"=w1748:refnum<class "Acquisition.lvclass">, "S4ACS_GUI out"=w1744:refnum<class "S4GUI.lvclass">)  [unwired: 7 in]
          n681 = call-dynamic "Read Channel.vi"("error in (no error)"=w1747, "Acquisition in"=w1748) -> ("error out"=w1739:errorcluster, "Channel.lvclass"=w1738:refnum<class "Channel.lvclass">, "Acquisition out"=w1746:refnum<class "Acquisition.lvclass">)  [unwired: 7 in]
          n682 = call-dynamic "Read State Machine.vi"("error in (no error)"=w1739, "Device in"=w1738) -> ("error out"=w1730:errorcluster, "State Machine.lvclass"=w1732:refnum<class "State Machine.lvclass">, "Device out"=w1736:refnum<class "Channel.lvclass">)  [unwired: 7 in]
          n683 = call-dynamic "Read State.vi"("error in (no error)"=w1730, "State Machine in"=w1732) -> ("error out"=w1729:errorcluster, "State"=w1726:i32, "State Machine out"=w1731:refnum<class "State Machine.lvclass">)  [unwired: 7 in]
          n684 = Equal To 0?(x=w1726) -> (x = 0?=w1728:bool)
          n685 = call-dynamic "Write State Machine.vi"("error in (no error)"=w1729, "State Machine.lvclass"=w1731, "Device in"=w1736) -> ("error out"=w1735:errorcluster, "Device out"=w1737:refnum<class "Channel.lvclass">)  [unwired: 7 in]
          n686 = call-dynamic "Write Channel.vi"("error in (no error)"=w1735, "Channel.lvclass"=w1737, "Acquisition in"=w1746) -> ("error out"=w1743:errorcluster, "Acquisition out"=w1745:refnum<class "Acquisition.lvclass">)  [unwired: 7 in]
          n687 = Select(t=u32 299, s=w1728, f=w1725) -> (s? t:f=w1727:u32)
          n688 = call-dynamic "Write AcquisitionD.vi"("error in (no error)"=w1743, "Acquisition.lvclass"=w1745, "S4ACS_GUI in"=w1744) -> ("error out"=w1740:errorcluster, "S4ACS_GUI out"=w1734:refnum<class "S4GUI.lvclass">)  [unwired: 7 in]
          n689 = Bundle By Name(cluster=w1734, "Obs_state"=w1727) -> (w1733:refnum<class "S4GUI.lvclass">)
        }
        frame 271 {
          # "Prepara os canais de aquisição para sequencia de foco...."
          n690 = flat-sequence {
            tunnel: w1775 -> [w1880]
            tunnel: [w1880] -> w1774
            frame #0 {
              n691 = Tick Count (ms)() -> (millisecond timer value=→"time5":u32)
            }
          }
          n692 = call-dynamic "Read AcquisitionA.vi"("error in (no error)"=w1774, "S4ACS_GUI in"=w1796) -> ("error out"=w1794:errorcluster, "Acquisition.lvclass"=w1795:refnum<class "Acquisition.lvclass">, "S4ACS_GUI out"=w1798:refnum<class "S4GUI.lvclass">)  [unwired: 7 in]
          n693 = call "Read connection.vi"("error in (no error)"=w1794, "Server in"=w1795) -> ("error out"=w1793:errorcluster, "connection"=w1773:bool, "Server out"=w1792:refnum<class "Acquisition.lvclass">)  [unwired: 7 in]
          n694 = case shown="True" w1773 {
            tunnel: [w1861 w1879] -> w1799
            tunnel: [w1860 w1878] -> w1797
            tunnel: w1793 -> [w1860 w1877]
            tunnel: w1792 -> [w1861 w1876]
            frame False {
            }
            frame True {
              # "configura o canal,\nmas não dispara\na exposicao."
              n695 = call-dynamic "Read Channel.vi"("error in (no error)"=w1877, "Acquisition in"=w1876) -> ("error out"=w1866:errorcluster, "Channel.lvclass"=w1868:refnum<class "Channel.lvclass">, "Acquisition out"=w1875:refnum<class "Acquisition.lvclass">)  [unwired: 7 in]
              n696 = call-dynamic "Write expose.vi"("error in (no error)"=w1866, "expose"=FALSE, "Channel in"=w1868) -> ("error out"=w1865:errorcluster, "Channel out"=w1867:refnum<class "Channel.lvclass">)  [unwired: 7 in]
              n697 = call-dynamic "Read State Machine.vi"("error in (no error)"=w1865, "Device in"=w1867) -> ("error out"=w1872:errorcluster, "State Machine.lvclass"=w1874:refnum<class "State Machine.lvclass">, "Device out"=w1870:refnum<class "Channel.lvclass">)  [unwired: 7 in]
              n698 = call "Next State.vi"("error in (no error)"=w1872, "New_State"=1, "State Machine in"=w1874) -> ("error out"=w1862:errorcluster, "State Machine out"=w1863:refnum<class "State Machine.lvclass">)  [unwired: 7 in]
              n699 = call-dynamic "Write State Machine.vi"("error in (no error)"=w1862, "State Machine.lvclass"=w1863, "Device in"=w1870) -> ("error out"=w1869:errorcluster, "Device out"=w1871:refnum<class "Channel.lvclass">)  [unwired: 7 in]
              n700 = call-dynamic "Write Channel.vi"("error in (no error)"=w1869, "Channel.lvclass"=w1871, "Acquisition in"=w1875) -> ("error out"=w1878:errorcluster, "Acquisition out"=w1879:refnum<class "Acquisition.lvclass">)  [unwired: 7 in]
            }
          }
          n701 = Increment(x=w1791) -> (x+1=w1755:u32)
          n702 = call-dynamic "Write AcquisitionA.vi"("error in (no error)"=w1797, "Acquisition.lvclass"=w1799, "S4ACS_GUI in"=w1798) -> ("error out"=w1787:errorcluster, "S4ACS_GUI out"=w1786:refnum<class "S4GUI.lvclass">)  [unwired: 7 in]
          n703 = call "Read AcquisitionB.vi"("error in (no error)"=w1787, "S4ACS_GUI in"=w1786) -> ("error out"=w1788:errorcluster, "Acquisition.lvclass"=w1789:refnum<class "Acquisition.lvclass">, "S4ACS_GUI out"=w1790:refnum<class "S4GUI.lvclass">)  [unwired: 7 in]
          n704 = call "Read connection.vi"("error in (no error)"=w1788, "Server in"=w1789) -> ("error out"=w1771:errorcluster, "connection"=w1770:bool, "Server out"=w1772:refnum<class "Acquisition.lvclass">)  [unwired: 7 in]
          n705 = case shown="True" w1770 {
            tunnel: [w1841 w1859] -> w1769
            tunnel: [w1840 w1858] -> w1768
            tunnel: w1771 -> [w1840 w1857]
            tunnel: w1772 -> [w1841 w1856]
            frame False {
            }
            frame True {
              # "configura o canal,\nmas não dispara\na exposicao."
              n706 = call-dynamic "Read Channel.vi"("error in (no error)"=w1857, "Acquisition in"=w1856) -> ("error out"=w1846:errorcluster, "Channel.lvclass"=w1848:refnum<class "Channel.lvclass">, "Acquisition out"=w1855:refnum<class "Acquisition.lvclass">)  [unwired: 7 in]
              n707 = call-dynamic "Write expose.vi"("error in (no error)"=w1846, "expose"=FALSE, "Channel in"=w1848) -> ("error out"=w1845:errorcluster, "Channel out"=w1847:refnum<class "Channel.lvclass">)  [unwired: 7 in]
              n708 = call-dynamic "Read State Machine.vi"("error in (no error)"=w1845, "Device in"=w1847) -> ("error out"=w1852:errorcluster, "State Machine.lvclass"=w1854:refnum<class "State Machine.lvclass">, "Device out"=w1850:refnum<class "Channel.lvclass">)  [unwired: 7 in]
              n709 = call "Next State.vi"("error in (no error)"=w1852, "New_State"=1, "State Machine in"=w1854) -> ("error out"=w1842:errorcluster, "State Machine out"=w1843:refnum<class "State Machine.lvclass">)  [unwired: 7 in]
              n710 = call-dynamic "Write State Machine.vi"("error in (no error)"=w1842, "State Machine.lvclass"=w1843, "Device in"=w1850) -> ("error out"=w1849:errorcluster, "Device out"=w1851:refnum<class "Channel.lvclass">)  [unwired: 7 in]
              n711 = call-dynamic "Write Channel.vi"("error in (no error)"=w1849, "Channel.lvclass"=w1851, "Acquisition in"=w1855) -> ("error out"=w1858:errorcluster, "Acquisition out"=w1859:refnum<class "Acquisition.lvclass">)  [unwired: 7 in]
            }
          }
          n712 = call "Write AcquisitionB.vi"("error in (no error)"=w1768, "Acquisition.lvclass"=w1769, "S4ACS_GUI in"=w1790) -> ("error out"=w1779:errorcluster, "S4ACS_GUI out"=w1778:refnum<class "S4GUI.lvclass">)  [unwired: 7 in]
          n713 = call-dynamic "Read AcquisitionC.vi"("error in (no error)"=w1779, "S4ACS_GUI in"=w1778) -> ("error out"=w1783:errorcluster, "Acquisition.lvclass"=w1784:refnum<class "Acquisition.lvclass">, "S4ACS_GUI out"=w1785:refnum<class "S4GUI.lvclass">)  [unwired: 7 in]
          n714 = call "Read connection.vi"("error in (no error)"=w1783, "Server in"=w1784) -> ("error out"=w1765:errorcluster, "connection"=w1766:bool, "Server out"=w1767:refnum<class "Acquisition.lvclass">)  [unwired: 7 in]
          n715 = case shown="True" w1766 {
            tunnel: [w1821 w1839] -> w1764
            tunnel: [w1820 w1838] -> w1763
            tunnel: w1765 -> [w1820 w1837]
            tunnel: w1767 -> [w1821 w1836]
            frame False {
            }
            frame True {
              # "configura o canal,\nmas não dispara\na exposicao."
              n716 = call-dynamic "Read Channel.vi"("error in (no error)"=w1837, "Acquisition in"=w1836) -> ("error out"=w1826:errorcluster, "Channel.lvclass"=w1828:refnum<class "Channel.lvclass">, "Acquisition out"=w1835:refnum<class "Acquisition.lvclass">)  [unwired: 7 in]
              n717 = call-dynamic "Write expose.vi"("error in (no error)"=w1826, "expose"=FALSE, "Channel in"=w1828) -> ("error out"=w1825:errorcluster, "Channel out"=w1827:refnum<class "Channel.lvclass">)  [unwired: 7 in]
              n718 = call-dynamic "Read State Machine.vi"("error in (no error)"=w1825, "Device in"=w1827) -> ("error out"=w1832:errorcluster, "State Machine.lvclass"=w1834:refnum<class "State Machine.lvclass">, "Device out"=w1830:refnum<class "Channel.lvclass">)  [unwired: 7 in]
              n719 = call "Next State.vi"("error in (no error)"=w1832, "New_State"=1, "State Machine in"=w1834) -> ("error out"=w1822:errorcluster, "State Machine out"=w1823:refnum<class "State Machine.lvclass">)  [unwired: 7 in]
              n720 = call-dynamic "Write State Machine.vi"("error in (no error)"=w1822, "State Machine.lvclass"=w1823, "Device in"=w1830) -> ("error out"=w1829:errorcluster, "Device out"=w1831:refnum<class "Channel.lvclass">)  [unwired: 7 in]
              n721 = call-dynamic "Write Channel.vi"("error in (no error)"=w1829, "Channel.lvclass"=w1831, "Acquisition in"=w1835) -> ("error out"=w1838:errorcluster, "Acquisition out"=w1839:refnum<class "Acquisition.lvclass">)  [unwired: 7 in]
            }
          }
          n722 = call-dynamic "Write AcquisitionC.vi"("error in (no error)"=w1763, "Acquisition.lvclass"=w1764, "S4ACS_GUI in"=w1785) -> ("error out"=w1777:errorcluster, "S4ACS_GUI out"=w1776:refnum<class "S4GUI.lvclass">)  [unwired: 7 in]
          n723 = call-dynamic "Read AcquisitionD.vi"("error in (no error)"=w1777, "S4ACS_GUI in"=w1776) -> ("error out"=w1780:errorcluster, "Acquisition.lvclass"=w1781:refnum<class "Acquisition.lvclass">, "S4ACS_GUI out"=w1782:refnum<class "S4GUI.lvclass">)  [unwired: 7 in]
          n724 = call "Read connection.vi"("error in (no error)"=w1780, "Server in"=w1781) -> ("error out"=w1760:errorcluster, "connection"=w1762:bool, "Server out"=w1761:refnum<class "Acquisition.lvclass">)  [unwired: 7 in]
          n725 = case shown="True" w1762 {
            tunnel: [w1801 w1819] -> w1759
            tunnel: [w1800 w1818] -> w1758
            tunnel: w1760 -> [w1800 w1817]
            tunnel: w1761 -> [w1801 w1816]
            frame False {
            }
            frame True {
              # "configura o canal,\nmas não dispara\na exposicao."
              n726 = call-dynamic "Read Channel.vi"("error in (no error)"=w1817, "Acquisition in"=w1816) -> ("error out"=w1806:errorcluster, "Channel.lvclass"=w1808:refnum<class "Channel.lvclass">, "Acquisition out"=w1815:refnum<class "Acquisition.lvclass">)  [unwired: 7 in]
              n727 = call-dynamic "Write expose.vi"("error in (no error)"=w1806, "expose"=FALSE, "Channel in"=w1808) -> ("error out"=w1805:errorcluster, "Channel out"=w1807:refnum<class "Channel.lvclass">)  [unwired: 7 in]
              n728 = call-dynamic "Read State Machine.vi"("error in (no error)"=w1805, "Device in"=w1807) -> ("error out"=w1812:errorcluster, "State Machine.lvclass"=w1814:refnum<class "State Machine.lvclass">, "Device out"=w1810:refnum<class "Channel.lvclass">)  [unwired: 7 in]
              n729 = call "Next State.vi"("error in (no error)"=w1812, "New_State"=1, "State Machine in"=w1814) -> ("error out"=w1802:errorcluster, "State Machine out"=w1803:refnum<class "State Machine.lvclass">)  [unwired: 7 in]
              n730 = call-dynamic "Write State Machine.vi"("error in (no error)"=w1802, "State Machine.lvclass"=w1803, "Device in"=w1810) -> ("error out"=w1809:errorcluster, "Device out"=w1811:refnum<class "Channel.lvclass">)  [unwired: 7 in]
              n731 = call-dynamic "Write Channel.vi"("error in (no error)"=w1809, "Channel.lvclass"=w1811, "Acquisition in"=w1815) -> ("error out"=w1818:errorcluster, "Acquisition out"=w1819:refnum<class "Acquisition.lvclass">)  [unwired: 7 in]
            }
          }
          n732 = call-dynamic "Write AcquisitionD.vi"("error in (no error)"=w1758, "Acquisition.lvclass"=w1759, "S4ACS_GUI in"=w1782) -> ("error out"=w1750:errorcluster, "S4ACS_GUI out"=w1754:refnum<class "S4GUI.lvclass">)  [unwired: 7 in]
          n733 = Unbundle By Name(w1754) -> ("TelFocus.lvclass"=w1753:refnum<class "TelFocus.lvclass">)
          n734 = call-dynamic "Write focus #stepsdone.vi"("error in (no error)"=w1750, "focus #stepsdone"=u32 0, "TelFocus in"=w1753) -> ("error out"=w1749:errorcluster, "TelFocus out"=w1751:refnum<class "TelFocus.lvclass">)  [unwired: 7 in]
          n735 = Bundle By Name(cluster=w1754, "TelFocus.lvclass"=w1751, "Error Msg"="", "Obs_state"=w1755) -> (w1756:refnum<class "S4GUI.lvclass">)
        }
        frame 272 {
          w1890 = 38 ("x")
          w1899 = 28 ("x")
          # "Se algum canal foi pra 38: Texp inválido \npara a configuração do CCD."
          # "Se algum canal foi pra 28: ERRO na inicialização."
          # "Espera terminar a execução da preparação\ndos 4 canais antes de ir ao proximo passo \nda Observação."
          n736 = flat-sequence {
            tunnel: w1932 -> [w2037]
            tunnel: [w2037] -> w1931
            frame #0 {
              n737 = Tick Count (ms)() -> (millisecond timer value=→"time6":u32)
            }
          }
          n738 = call-dynamic "Read AcquisitionA.vi"("error in (no error)"=w1931, "S4ACS_GUI in"=w1942) -> ("error out"=w1929:errorcluster, "Acquisition.lvclass"=w1930:refnum<class "Acquisition.lvclass">, "S4ACS_GUI out"=w1944:refnum<class "S4GUI.lvclass">)  [unwired: 7 in]
          n739 = call "Read connection.vi"("error in (no error)"=w1929, "Server in"=w1930) -> ("error out"=w1927:errorcluster, "connection"=w1926:bool, "Server out"=w1928:refnum<class "Acquisition.lvclass">)  [unwired: 7 in]
          n740 = case shown="True" w1926 {
            tunnel: w1928 -> [w2020 w2036]
            tunnel: w1927 -> [w2019 w2035]
            tunnel: [w2020 w2033] -> w1945
            tunnel: [w2019 w2032] -> w1943
            tunnel: [0 ("State") w2022] -> w1889
            frame False {
            }
            frame True {
              n741 = call-dynamic "Read Channel.vi"("error in (no error)"=w2035, "Acquisition in"=w2036) -> ("error out"=w2031:errorcluster, "Channel.lvclass"=w2030:refnum<class "Channel.lvclass">, "Acquisition out"=w2034:refnum<class "Acquisition.lvclass">)  [unwired: 7 in]
              n742 = call-dynamic "Read State Machine.vi"("error in (no error)"=w2031, "Device in"=w2030) -> ("error out"=w2024:errorcluster, "State Machine.lvclass"=w2026:refnum<class "State Machine.lvclass">, "Device out"=w2028:refnum<class "Channel.lvclass">)  [unwired: 7 in]
              n743 = call-dynamic "Read State.vi"("error in (no error)"=w2024, "State Machine in"=w2026) -> ("error out"=w2023:errorcluster, "State"=w2022:i32, "State Machine out"=w2025:refnum<class "State Machine.lvclass">)  [unwired: 7 in]
              n744 = call-dynamic "Write State Machine.vi"("error in (no error)"=w2023, "State Machine.lvclass"=w2025, "Device in"=w2028) -> ("error out"=w2027:errorcluster, "Device out"=w2029:refnum<class "Channel.lvclass">)  [unwired: 7 in]
              n745 = call-dynamic "Write Channel.vi"("error in (no error)"=w2027, "Channel.lvclass"=w2029, "Acquisition in"=w2034) -> ("error out"=w2032:errorcluster, "Acquisition out"=w2033:refnum<class "Acquisition.lvclass">)  [unwired: 7 in]
            }
          }
          n746 = call-dynamic "Write AcquisitionA.vi"("error in (no error)"=w1943, "Acquisition.lvclass"=w1945, "S4ACS_GUI in"=w1944) -> ("error out"=w1939:errorcluster, "S4ACS_GUI out"=w1938:refnum<class "S4GUI.lvclass">)  [unwired: 7 in]
          n747 = call "Read AcquisitionB.vi"("error in (no error)"=w1939, "S4ACS_GUI in"=w1938) -> ("error out"=w1921:errorcluster, "Acquisition.lvclass"=w1924:refnum<class "Acquisition.lvclass">, "S4ACS_GUI out"=w1925:refnum<class "S4GUI.lvclass">)  [unwired: 7 in]
          n748 = call "Read connection.vi"("error in (no error)"=w1921, "Server in"=w1924) -> ("error out"=w1920:errorcluster, "connection"=w1922:bool, "Server out"=w1923:refnum<class "Acquisition.lvclass">)  [unwired: 7 in]
          n749 = case shown="True" w1922 {
            tunnel: w1923 -> [w2002 w2018]
            tunnel: w1920 -> [w2001 w2017]
            tunnel: [w2002 w2015] -> w1919
            tunnel: [w2001 w2014] -> w1918
            tunnel: [0 ("State") w2004] -> w1888
            frame False {
            }
            frame True {
              n750 = call-dynamic "Read Channel.vi"("error in (no error)"=w2017, "Acquisition in"=w2018) -> ("error out"=w2013:errorcluster, "Channel.lvclass"=w2012:refnum<class "Channel.lvclass">, "Acquisition out"=w2016:refnum<class "Acquisition.lvclass">)  [unwired: 7 in]
              n751 = call-dynamic "Read State Machine.vi"("error in (no error)"=w2013, "Device in"=w2012) -> ("error out"=w2006:errorcluster, "State Machine.lvclass"=w2008:refnum<class "State Machine.lvclass">, "Device out"=w2010:refnum<class "Channel.lvclass">)  [unwired: 7 in]
              n752 = call-dynamic "Read State.vi"("error in (no error)"=w2006, "State Machine in"=w2008) -> ("error out"=w2005:errorcluster, "State"=w2004:i32, "State Machine out"=w2007:refnum<class "State Machine.lvclass">)  [unwired: 7 in]
              n753 = call-dynamic "Write State Machine.vi"("error in (no error)"=w2005, "State Machine.lvclass"=w2007, "Device in"=w2010) -> ("error out"=w2009:errorcluster, "Device out"=w2011:refnum<class "Channel.lvclass">)  [unwired: 7 in]
              n754 = call-dynamic "Write Channel.vi"("error in (no error)"=w2009, "Channel.lvclass"=w2011, "Acquisition in"=w2016) -> ("error out"=w2014:errorcluster, "Acquisition out"=w2015:refnum<class "Acquisition.lvclass">)  [unwired: 7 in]
            }
          }
          n755 = call "Write AcquisitionB.vi"("error in (no error)"=w1918, "Acquisition.lvclass"=w1919, "S4ACS_GUI in"=w1925) -> ("error out"=w1937:errorcluster, "S4ACS_GUI out"=w1936:refnum<class "S4GUI.lvclass">)  [unwired: 7 in]
          n756 = call-dynamic "Read AcquisitionC.vi"("error in (no error)"=w1937, "S4ACS_GUI in"=w1936) -> ("error out"=w1916:errorcluster, "Acquisition.lvclass"=w1917:refnum<class "Acquisition.lvclass">, "S4ACS_GUI out"=w1941:refnum<class "S4GUI.lvclass">)  [unwired: 7 in]
          n757 = call "Read connection.vi"("error in (no error)"=w1916, "Server in"=w1917) -> ("error out"=w1915:errorcluster, "connection"=w1913:bool, "Server out"=w1914:refnum<class "Acquisition.lvclass">)  [unwired: 7 in]
          n758 = case shown="True" w1913 {
            tunnel: w1914 -> [w1984 w2000]
            tunnel: w1915 -> [w1983 w1999]
